vi "Resolve UI Dependencies.vi"(8 "error in":errorcluster, 11 "Template Project Path":path) -> (0 "error out":errorcluster)   [LabVIEW 2021, in "Plugin Generator.lvlib"]
uses:
  Plugin Generator.lvlib
  <vilib>/Utility/traverseref.llb/VI Scripting - Traverse.lvlib
  <vilib>/Utility/traverseref.llb/TRef TravTarget.ctl
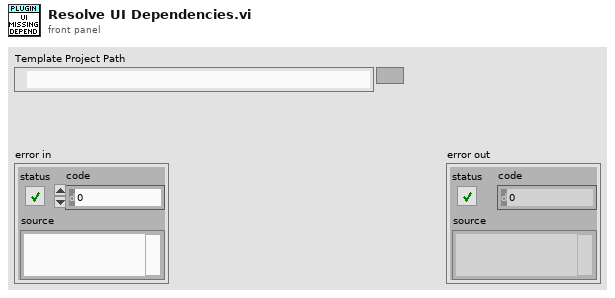
[diagram p1: front panel]
types:
  T1 = typedef "TRef TravTarget.ctl" = enum16{"FP", "BD", "Other"}
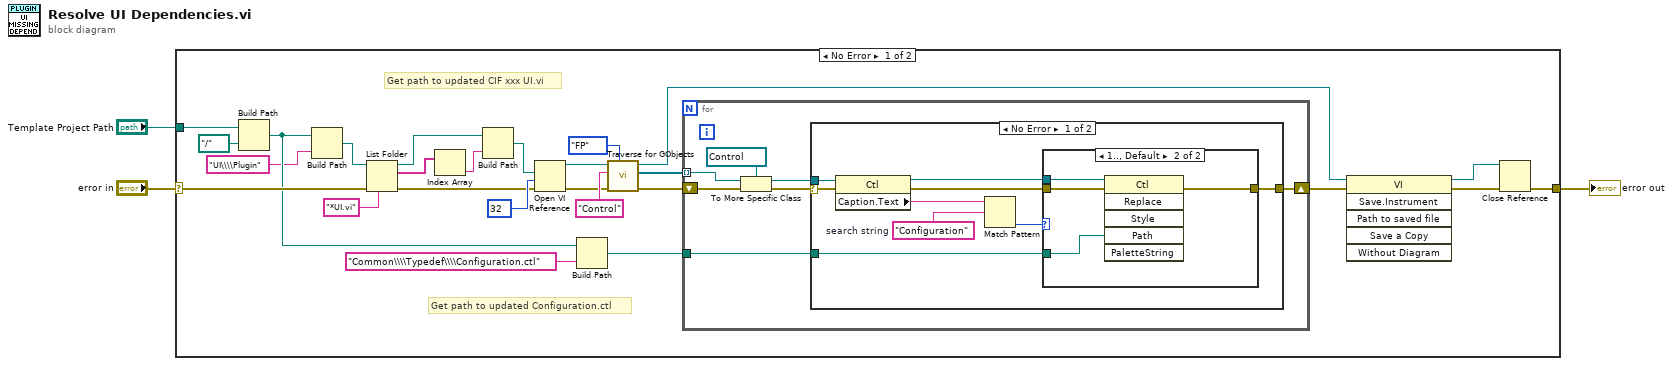
[diagram p0: block diagram]
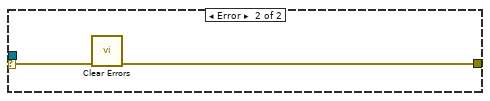
[diagram p3: hidden frame]
diagram:
  n1 = case shown="No Error" "error in" {
    selector: "error in" -> [w26 w53]
    tunnel: [w11 w53] -> w3
    tunnel: "Template Project Path" -> [w29 _]
    frame No Error {
      # "Get path to updated Configuration.ctl"
      # "Get path to updated CIF xxx UI.vi"
      n2 = Build Path(base path=w29, name or relative path=path "../..") -> (appended path=w9:path)
      n3 = Build Path(base path=w9, name or relative path="UI\\\\Plugin" ("Class Name")) -> (appended path=w27:path)
      n4 = List Folder(path=w27, pattern="*UI.vi" ("Class Name"), error in=w26) -> (path out=w25:path, filenames=w24:string[], error out=w7:errorcluster)  [unwired: 1 in, 1 out]
      n5 = Index Array(array=w24) -> (element=w23:string)  [unwired: 1 in]
      n6 = Build Path(base path=w25, name or relative path=w23) -> (appended path=w6:path)
      n7 = Open VI Reference(vi path=w6, options=32, error in (no error)=w7) -> (vi reference=w10:refnum<vi>, error out=w8:errorcluster)  [unwired: 3 in]
      n8 = Build Path(base path=w9, name or relative path="Common\\\\Typedef\\\\Configuration.ctl" ("Class Name")) -> (appended path=w16:path)
      n9 = call <vilib>:"Traverse for GObjects.vi"("Traverse Target"=TRef_TravTarget."FP", "error in (no error)"=w8, "Class Name"="Control", "VI Refnum"=w10) -> ("error out"=w17:errorcluster, "References"=w20:refnum<vi>[], "dup VI Refnum"=w4:refnum<vi>)  [unwired: 4 in, 1 out]
      n10 = for {
        tunnel: w20 -> [w36] mode=indexing
        shift-right: [w34] -> w15
        shift-left: w17 -> [w32]
        tunnel: w16 -> [w31]
        n11 = To More Specific Class(target class=refnum<vi> refnum ("x"), reference=w36, error in=w32) -> (specific class reference=w33:refnum<vi>, error out=w30:errorcluster)
        n12 = case shown="No Error" w30 {
          selector: w30 -> [w37 w52]
          tunnel: [w43 w51] -> w34
          tunnel: w33 -> [w42 _]
          tunnel: w31 -> [w40 _]
          frame No Error {
            w39 = "Configuration"  # search string
            n13 = property class="Ctl"(reference=w42, error in=w37) -> (reference out=w44:refnum<vi>, error out=w45:errorcluster, "Caption.Text"=w41:string)
            n14 = Match Pattern(string=w41, regular expression=w39) -> (offset past match=w38:i32)  [unwired: 1 in, 3 out]
            n15 = case shown="1.., Default" w38 {
              tunnel: w45 -> [w46 w48]
              tunnel: w44 -> [_ w47]
              tunnel: [w46 w50] -> w43
              tunnel: w40 -> [_ w49]
              frame -1 {
              }
              frame 1.., Default {
                n16 = invoke class="Ctl" method="Replace"(reference=w47, error in=w48, "Path"=w49) -> (error out=w50:errorcluster)  [unwired: 3 in, 5 out]
              }
            }
          }
          frame Error {
            n17 = call <vilib>:"Clear Errors.vi"("error in (no error)"=w52) -> ("error out"=w51:errorcluster)  [unwired: 5 in, 1 out]
          }
        }
      }
      n18 = invoke class="VI" method="Save.Instrument"(reference=w4, error in=w15) -> (reference out=w12:refnum<vi>, error out=w13:errorcluster)  [unwired: 4 in, 4 out]
      n19 = Close Reference(reference=w12, error in (no error)=w13) -> (error out=w11:errorcluster)
    }
    frame Error {
    }
  }
  "error out" <- w3
